vi "Read TDMS Wave 1D.vi"(4 "Append Index":i32, 8 "error in (no error)":errorcluster, 10 "channel name(s) in":string, 11 "path":path) -> (0 "error out":errorcluster, 2 "data":dbl[](array[numeric]), 3 "file path out":path)   [LabVIEW 2016, in "Data.TDMS.lvclass"]
uses:
  Data.TDMS.lvclass
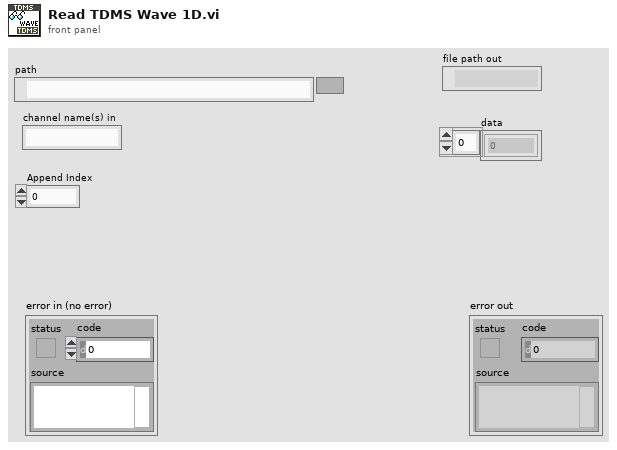
[diagram p1: front panel]
types:
  T1 = enum16{"open", "open or create", "create or replace", "create", "open (read-only)"}
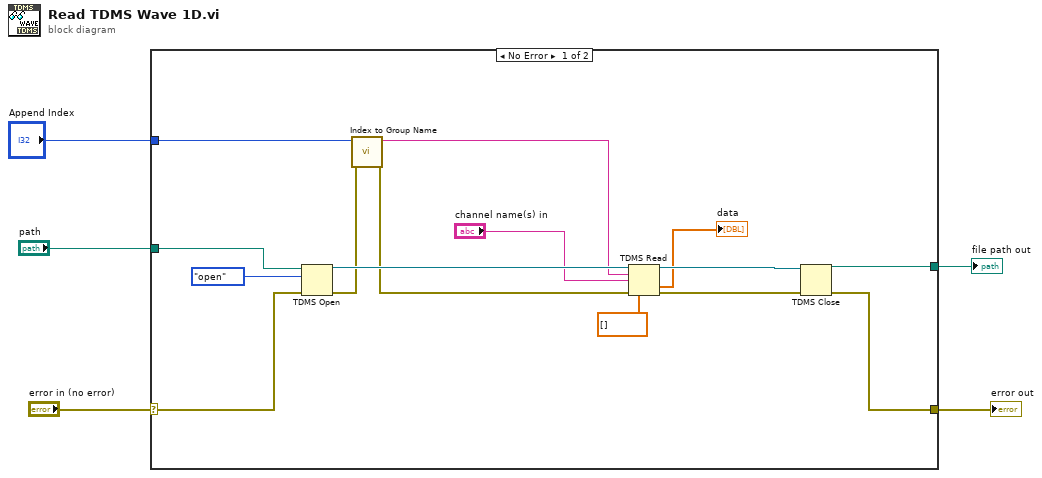
[diagram p0: block diagram]
diagram:
  n1 = case shown="No Error" "error in (no error)" {
    selector: "error in (no error)" -> [w11 w21]
    tunnel: [w19 w21] -> w4
    tunnel: "path" -> [w16 _]
    tunnel: [w10 _] -> w2
    tunnel: "Append Index" -> [w6 _]
    frame No Error {
      n2 = TDMS Open(8:w11, 10:T1."open" ("operation (0:open)"), 11:w16) -> (0:w8:errorcluster, 3:w14:refnum<k34>)  [unwired: 4 in]
      n3 = call "Index to Group Name.vi"("error in (no error)"=w8, "Append Index"=w6) -> ("error out"=w7:errorcluster, "group name in (Untitled)"=w9:string)  [unwired: 8 in]
      n4 = TDMS Read(0:w14, 5:w9, 7:"channel name(s) in", 11:w7, 12:dbl[] [] ("array type (2D Dbl)")) -> (4:w18:refnum<k34>, 10:→"data":dbl[], 15:w17:errorcluster)  [unwired: 3 in, 3 out]
      n5 = TDMS Close(8:w17, 11:w18) -> (0:w19:errorcluster, 3:w10:path)
    }
    frame Error {
    }
  }
  "error out" <- w4
  "file path out" <- w2
